vi "Main VI FTP FILE MANAGER.vi"() -> ()   [LabVIEW 2011]
doc: "FILE Archive & FTP is a software used to handle the file management of remote field sites using the HTI Data Logger or ATR series acoustic equipment that generates *.RAT and *.ATL files. The software monitors a specific folder on the local machine that the HTI equipment has been set up to move completed files of these types into. All other file types are ignored. The software continues to scan this file until a new file is added to the directory, on the addition of a file the NODE ARCHIVE & FTP software moves the file into an Archive directory (and if specified into a redundant Archive directory) then creates a *.ZIP version of the file and retains a copy of it in the Archive directory as well. All Zip files are then copied to a specified FTP host.\n\nNODE ARCHIVE & FTP will not try and move files for the last five minutes of an hour, or for the first five to ten minutes of the hour (based on CPU time). This is to allow the HTI hardware time to move all files at the top of the hour and avoid conflict. During the rest of the hour the software will continue to scan for new files. At any time a user can force a scan or FTP move by selecting the Manual Force FTP button or the Manual Archive Files button.\n\nNODE ARCHIVE & FTP creates an .INI file and a .CSV file in the programs application directory. The .INI file retains the last values of the file directory and FTP credentials used. The .CSV retains a history of *.ZIP files moved to the FTP and the status of their move, if there were errors or not. NODE ARCHIVE & FTP will continue to try and send the file to the FTP host until that file has completed the process with no errors. DO NOT remove or edit the .CSV file or the software will try and move all files up to the FTP again and will slow down the FTP Host."
uses:
  Controls/FTP Credintials.ctl
  Controls/File Management.ctl
  Controls/File Path directories.ctl
  Controls/Ping address and email notify.ctl
  Controls/PingElements.ctl
  SubVIs/Bini ArchiveAndFtpCluster.ctl
  <vilib>/Utility/sysdir.llb/System Directory Type.ctl
panel:
  in  "SaveConfig":bool
  in  "Settings":bool
  in  "Contacts":bool
  in  "Errors":bool
  in  "SetPingStats":bool
  in  "Addresses to Ping":T1
  in  "File type Cover":bool
  in  "Auto Archive":bool
  in  "Auto FTP":bool
  in  "update extentions":bool
  in  "ShutDown":bool
  in  "FTP Creds":T2={"Host"="", "UserName"="", "PassWord"="", "FTP File Path"="", "Timeout (S)"=0, "ActivePasive"=FALSE, "Binary Ascii"=FALSE, "Remote Port"=21} {"Timeout (S)" min=0 max=300 step=1}
  in  "SITE ID":string="Site Not Configured" caption="Site ID:"
  in  "File Management":T3
  in  "Manual FTP":bool
  out "Archive in progress":bool caption="Archive"
  out "Status FTP move":bool caption="FTP"
  in  "Manual Archive":bool
  in  "File output directories":T4={"Archive Location"=path "", "Archive Location 2"=path "<Not A Path>", "OutPut Path"=path "", "Directory(s) To Scan Files"=[]}
  in  "time date mod":bool
  out "Elapsed Time (H)":dbl caption="Time since Last File \nSize Check (H)" format="%#_3f"
  in  "recipients":string[](array[string])=["nmswyers@gmail.com"] caption="Errors & Warnings Email Recipients"
  out "hours":u8
  out "Email Notification Cluster":T5
  in  "shutting down closeout":bool
  in  "Time DaY":timestamp
  # "D\nI\nR\nE\nC\nT\nO\nR\nY\n\nS\nE\nT"
  # "FILE \n\nHANDLE\n\nMETHODS"
  # "FTP\n\nSETUP"
  # "Passive"
  # "Active"
  # "Binary"
  # "Ascii"
  # "File Handling Method"
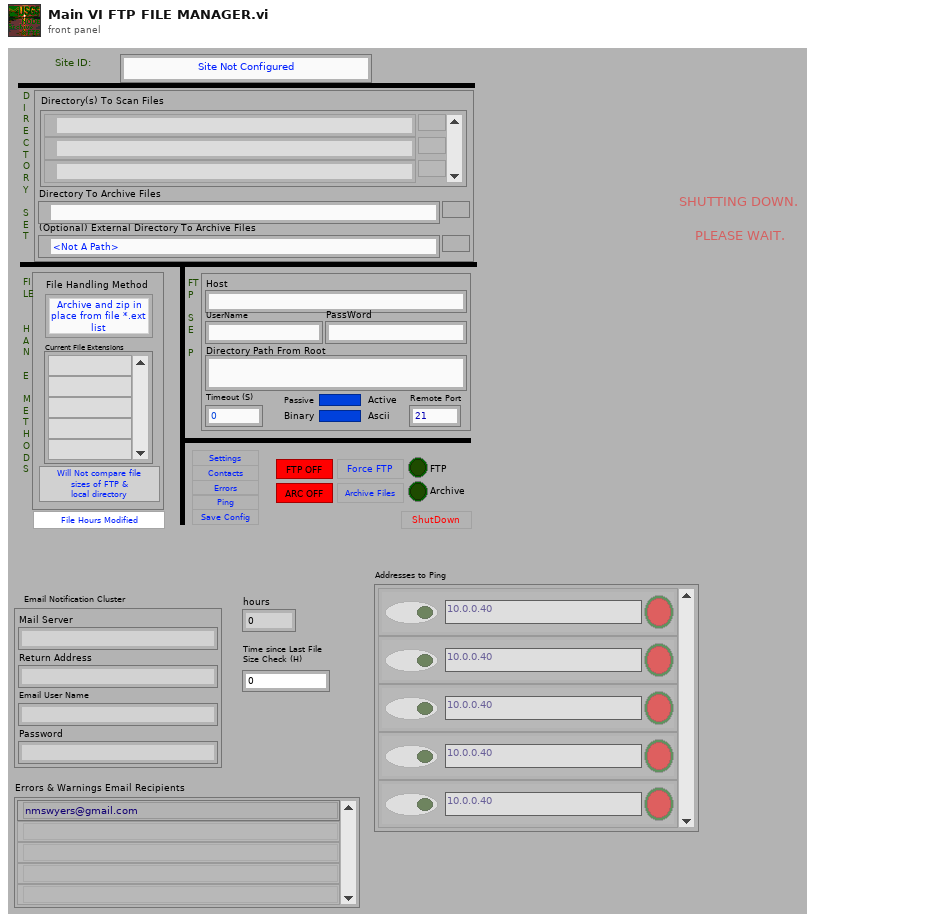
[diagram p1: front panel]
types:
  T1 = typedef "PingElements.ctl" = cluster{"AddressNode 1":string, "Response 1":bool, "Ping on Address 1":bool}[]
  T2 = typedef "FTP Credintials.ctl" = cluster{"Host":string, "UserName":string, "PassWord":string, "FTP File Path":string, "Timeout (S)":i32, "ActivePasive":bool, "Binary Ascii":bool, "Remote Port":u16}
  T3 = typedef "File Management.ctl" = cluster{"Comp File Size":bool, "File Handle Method":enum16{"Archive and zip in place from file *.ext list", "Archive and zip ALL file Types to archive directory", "Archive and zip to archive directory from file *.ext list", "Perform no file management"}, "file extention list":string[]}
  T4 = typedef "File Path directories.ctl" = cluster{"Archive Location":path, "Archive Location 2":path, "OutPut Path":path, "Directory(s) To Scan Files":path[]}
  T5 = typedef "Ping address and email notify.ctl" = cluster{"Mail Server":string, "Return Address":string, "Email User Name":string, "Password":string}
  T6 = enum16{"open", "replace", "create", "open or create", "replace or create", "replace or create with confirmation"}
  T7 = enum8{"Enabled", "Disabled", "Disabled and Grayed Out"}
  T8 = typedef "Bini ArchiveAndFtpCluster.ctl" = cluster{"Site ID":string, "File Management cluster":T3, "time stamp":timestamp, "File output directories":T4, "Auto FTP":bool, "Auto Archive":bool, "FTP CRED Cluster":T2, "hours old date mod(hours)":u8, "Email Notification Cluster":T5, "Email Recipiant List":string[], "Addresses to Ping":T1}
  T9 = enum16{"Archive and zip in place from file *.ext list", "Archive and zip ALL file Types to archive directory", "Archive and zip to archive directory from file *.ext list", "Perform no file management"}
  T10 = enum32{"Invalid", "Standard", "Closed", "Hidden", "Minimized", "Maximized"}
  T11 = cluster{"AddressNode 1":string, "Response 1":bool, "Ping on Address 1":bool}
  T12 = enum32{"invalid app kind", "Development System", "Run Time System", "Student Edition", "Embedded LabVIEW", "Evaluation", "Custom"}
  T13 = typedef "System Directory Type.ctl" = i32
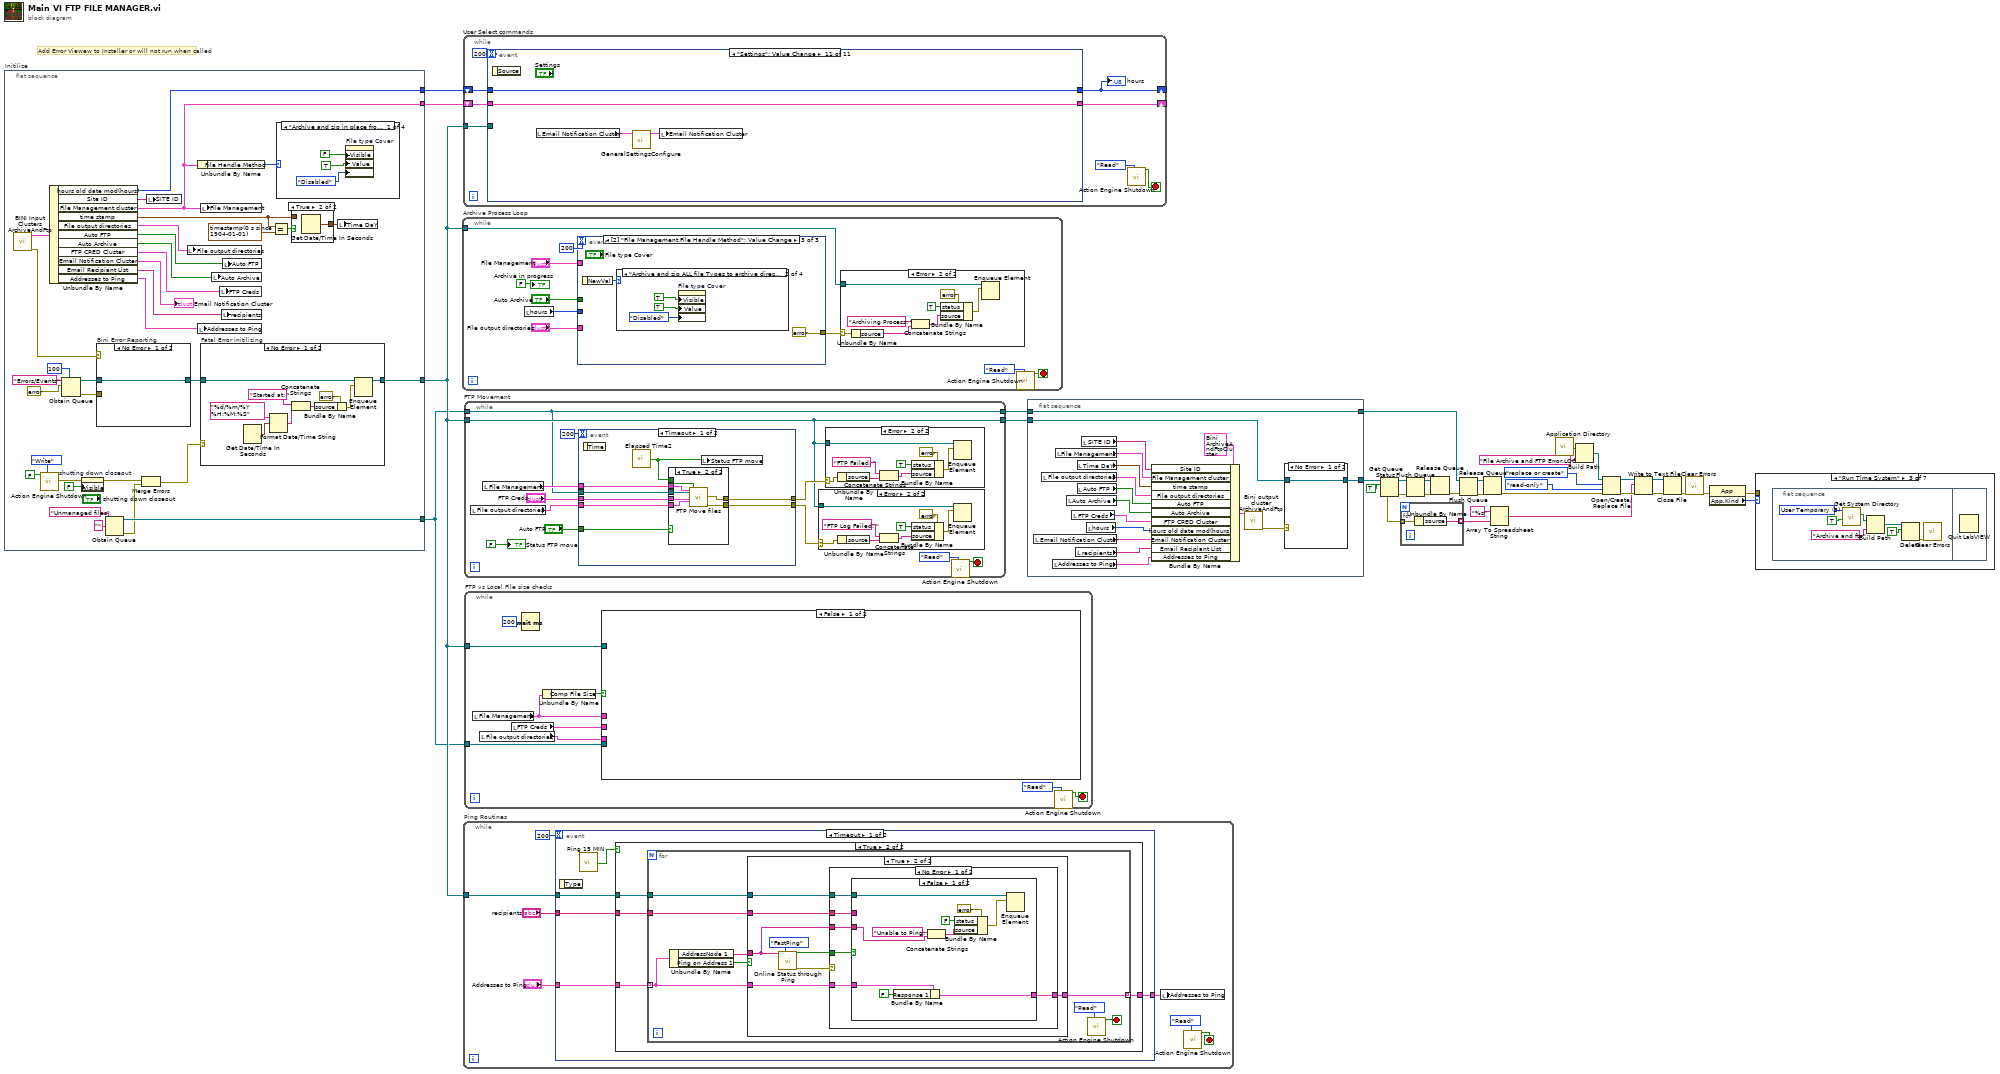
[diagram p0: block diagram]
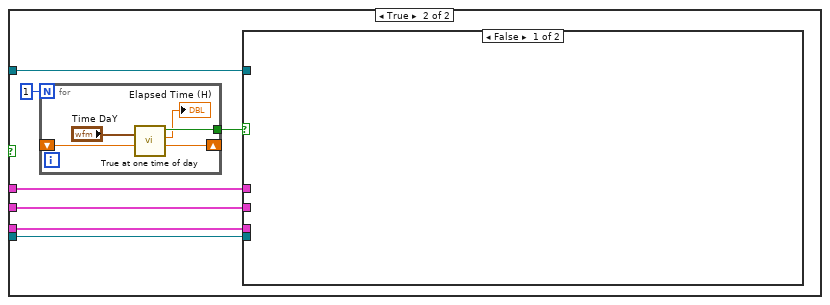
[diagram p2: hidden frame]
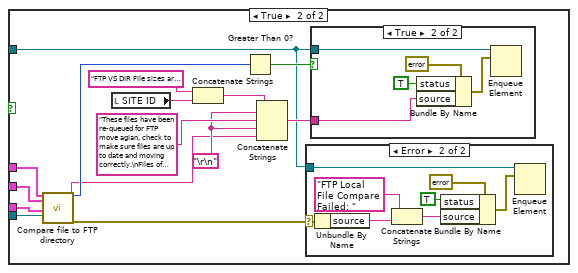
[diagram p3: hidden frame]
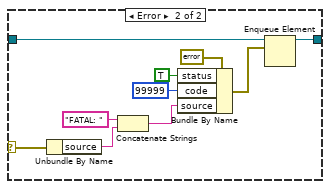
[diagram p7: hidden frame]
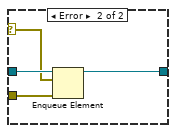
[diagram p8: hidden frame]
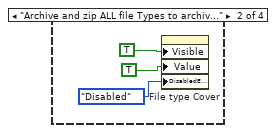
[diagram p9: hidden frame]
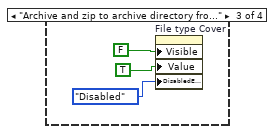
[diagram p10: hidden frame]
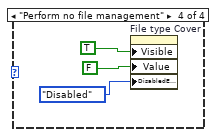
[diagram p11: hidden frame]
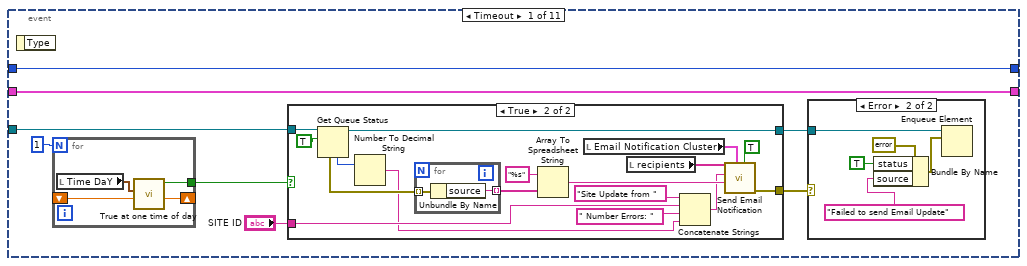
[diagram p12: hidden frame]
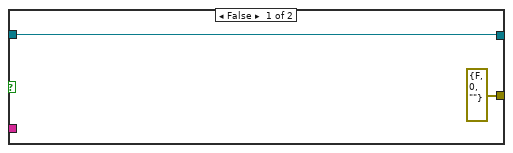
[diagram p14: hidden frame]
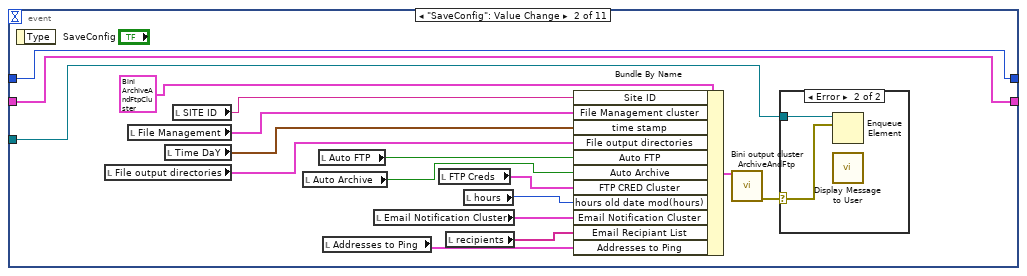
[diagram p15: hidden frame]
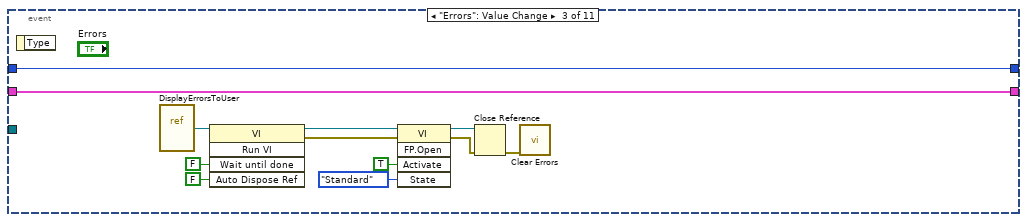
[diagram p17: hidden frame]
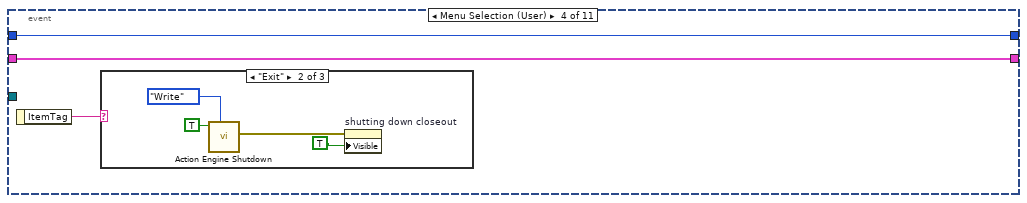
[diagram p18: hidden frame]
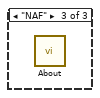
[diagram p20: hidden frame]
diagram:
  # "Add Error Viewew to Installer or will not run when called"
  n1 = flat-sequence "Initilize" {
    tunnel: [w66] -> w28
    tunnel: [w56] -> w31
    tunnel: [w51] -> w30
    tunnel: [w39] -> w29
    frame #0 {
      n2 = call "BINI Input Clusters ArchiveAndFtp.vi"() -> ("Bini Error out"=w46:errorcluster, "Bini Load"=w57:T8)  [unwired: 10 in]
      n3 = call "Action Engine Shutdown.vi"("Shutdown"=enum16{"Write", "Read"}."Write", "Shutdown (True to Shutdown)"=FALSE) -> ("error out"=w62:errorcluster)  [unwired: 8 in, 1 out]
      n4 = Unbundle By Name(w57) -> ("hours old date mod(hours)"=w51:u8, "Site ID"=w55:string, "File Management cluster"=w56:T3, "time stamp"=w35:timestamp, "File output directories"=w54:T4, "Auto FTP"=w53:bool, "Auto Archive"=w52:bool, "FTP CRED Cluster"=w50:T2, "Email Notification Cluster"=→"Email Notification Cluster":T5, "Email Recipiant List"=w48:string[], "Addresses to Ping"=w47:T1)
      n5 = Obtain Queue(max queue size (-1, unlimited)=100, name (unnamed)="Errors/Events", element data type=errorcluster {"status"=FALSE, "code"=0, "source"=""} ("error constant")) -> (queue out=w45:refnum<queue>, error out=w43:errorcluster)  [unwired: 2 in, 1 out]
      n6 = property on="shutting down closeout" class="Bool"(error in=w62, "Visible"=FALSE) -> (error out=w42:errorcluster)  [unwired: 1 in, 1 out]
      n7 = case "Bini Error Reporting" shown="No Error" w46 {
        selector: w46 -> [_ w92]
        tunnel: w45 -> [w90 w94]
        tunnel: [w90 w93] -> w40
        tunnel: w43 -> [_ w91]
        frame No Error {
        }
        frame Error {
          n8 = Enqueue Element(queue=w94, element=w92, error in (no error)=w91) -> (queue out=w93:refnum<queue>)  [unwired: 1 in, 2 out]
        }
      }
      n9 = Obtain Queue(name (unnamed)="Unmanaged files", element data type="" ("name (unnamed)")) -> (queue out=w66:refnum<queue>, error out=w60:errorcluster)  [unwired: 3 in, 1 out]
      n10 = Merge Errors(w42, w60) -> (w41:errorcluster)
      n11 = local write "SITE ID"(w55) -> ()
      n12 = local write "File output directories"(w54) -> ()
      n13 = Unbundle By Name(w56) -> ("File Handle Method"=w61:T9)
      n14 = local write "Addresses to Ping"(w47) -> ()
      n15 = local write "File Management"(w56) -> ()
      n16 = case "Fatal Error initilizing" shown="No Error" w41 {
        selector: w41 -> [_ w83]
        tunnel: w40 -> [w79 w89]
        tunnel: [w78 w88] -> w39
        frame No Error {
          n17 = Get Date/Time In Seconds() -> (seconds since 1Jan1904=w73:timestamp)
          n18 = Format Date/Time String(time format string (%c)="%d/%m/%Y %H:%M:%S", seconds (now)=w73) -> (date/time string=w72:string)  [unwired: 1 in]
          n19 = Concatenate Strings("Started at: " ("string"), w72) -> (w75:string)
          n20 = Bundle By Name(cluster=errorcluster {"status"=FALSE, "code"=0, "source"=""} ("element"), "source"=w75) -> (w76:errorcluster)
          n21 = Enqueue Element(queue=w79, element=w76) -> (queue out=w78:refnum<queue>)  [unwired: 2 in, 2 out]
        }
        frame Error {
          n22 = Unbundle By Name(w83) -> ("source"=w82:string)
          n23 = Concatenate Strings("FATAL: " ("string"), w82) -> (w85:string)
          n24 = Bundle By Name(cluster=errorcluster {"status"=FALSE, "code"=0, "source"=""} ("error constant"), "status"=TRUE, "code"=99999, "source"=w85) -> (w80:errorcluster)
          n25 = Enqueue Element(queue=w89, element=w80) -> (queue out=w88:refnum<queue>)  [unwired: 2 in, 2 out]
        }
      }
      n26 = local write "Auto Archive"(w52) -> ()
      n27 = local write "FTP Creds"(w50) -> ()
      n28 = local write "recipients"(w48) -> ()
      n29 = local write "Auto FTP"(w53) -> ()
      n30 = Equal?(x=w35, y=timestamp(0 s since 1904-01-01)) -> (x = y?=w38:bool)
      n31 = case shown="\"Archive and zip in place from file *.ext list\", Default" w61 {
        frame "Archive and zip in place from file *.ext list", Default {
          n32 = property on="File type Cover" class="Bool (strict)"("Visible"=FALSE, "Value"=TRUE ("File type Cover"), "DisabledEnum"=T7."Disabled" ("Disabled")) -> ()  [unwired: 2 in, 2 out]
        }
        frame "Archive and zip ALL file Types to archive directory" {
          n33 = property on="File type Cover" class="Bool (strict)"("Visible"=TRUE, "Value"=TRUE ("File type Cover"), "DisabledEnum"=T7."Disabled" ("Disabled")) -> ()  [unwired: 2 in, 2 out]
        }
        frame "Archive and zip to archive directory from file *.ext list" {
          n34 = property on="File type Cover" class="Bool (strict)"("Visible"=FALSE, "Value"=TRUE ("File type Cover"), "DisabledEnum"=T7."Disabled" ("Disabled")) -> ()  [unwired: 2 in, 2 out]
        }
        frame "Perform no file management" {
          n35 = property on="File type Cover" class="Bool (strict)"("Visible"=TRUE, "Value"=FALSE ("File type Cover"), "DisabledEnum"=T7."Disabled" ("Disabled")) -> ()  [unwired: 2 in, 2 out]
        }
      }
      n36 = case shown="True" w38 {
        tunnel: [w69 w70] -> w36
        tunnel: w35 -> [w69 _]
        frame False {
        }
        frame True {
          n37 = Get Date/Time In Seconds() -> (seconds since 1Jan1904=w70:timestamp)
        }
      }
      n38 = local write "Time DaY"(w36) -> ()
    }
  }
  n39 = while "Archive Process Loop" {
    tunnel: w29 -> [w107]
    stop <- w111 stop-if-true
    n40 = local read "hours"() -> (w108:u8)
    n41 = event shown="[2] \"File Management.File Handle Method\": Value Change" {
      selector: _ -> [_ _ _]
      dyn-events: _ -> [_ _ _]
      timeout: 200 -> [_ _ _]
      tunnel: [w130 w143 errorcluster {"status"=FALSE, "code"=0, "source"=""} ("error IO")] -> w110
      tunnel: "File output directories" -> [w125 w142 _]
      tunnel: "File Management" -> [w128 w140 _]
      tunnel: "Auto Archive" -> [w129 _ _]
      tunnel: w108 -> [w126 w139 _]
      event Timeout {
        n42 = event-data() -> ()  [unwired: 1 in, 1 out]
        n43 = call "Elapsed Time"() -> ("Time has Elapsed"=w127:bool)  [unwired: 12 in, 7 out]
        n44 = case shown="True" w129 {
          tunnel: w125 -> [w131 w138]
          tunnel: [errorcluster {"status"=FALSE, "code"=0, "source"=""} ("error IO") w137] -> w130
          tunnel: w128 -> [_ w136]
          tunnel: w127 -> [_ w135]
          tunnel: w126 -> [_ w134]
          tunnel: [w131 w133] -> _
          frame False {
          }
          frame True {
            n45 = call "Archive files move dir.vi"("hours old date mod(hours)"=w134, "File path input cluster"=w138, "File Management"=w136, "Timing True to archive"=w135) -> ("error IO"=w137:errorcluster, "File path input cluster (out)"=w133:T4)  [unwired: 4 in]
          }
        }
        n46 = local write "Archive in progress"(w127) -> ()
      }
      event "Manual Archive": Value Change {
        w141 = TRUE ("Status File move")
        n47 = event-data() -> ()  [unwired: 1 in, 1 out]
        n48 = local write "Archive in progress"(w141) -> ()
        n49 = call "Archive files move dir.vi"("hours old date mod(hours)"=w139, "File path input cluster"=w142, "File Management"=w140, "Timing True to archive"=w141) -> ("error IO"=w143:errorcluster)  [unwired: 4 in, 1 out]
      }
      event Value Change {
        n50 = event-data() -> ("NewVal"=w145:T9)  [unwired: 1 in]
        n51 = case shown="\"Archive and zip ALL file Types to archive directory\"" w145 {
          frame "Archive and zip in place from file *.ext list", Default {
            n52 = property on="File type Cover" class="Bool (strict)"("Visible"=FALSE, "Value"=TRUE ("File type Cover"), "DisabledEnum"=T7."Disabled" ("Disabled")) -> ()  [unwired: 2 in, 2 out]
          }
          frame "Archive and zip ALL file Types to archive directory" {
            n53 = property on="File type Cover" class="Bool (strict)"("Visible"=TRUE, "Value"=TRUE ("File type Cover"), "DisabledEnum"=T7."Disabled" ("Disabled")) -> ()  [unwired: 2 in, 2 out]
          }
          frame "Archive and zip to archive directory from file *.ext list" {
            n54 = property on="File type Cover" class="Bool (strict)"("Visible"=FALSE, "Value"=TRUE ("File type Cover"), "DisabledEnum"=T7."Disabled" ("Disabled")) -> ()  [unwired: 2 in, 2 out]
          }
          frame "Perform no file management" {
            n55 = property on="File type Cover" class="Bool (strict)"("Visible"=TRUE, "Value"=FALSE ("File type Cover"), "DisabledEnum"=T7."Disabled" ("Disabled")) -> ()  [unwired: 2 in, 2 out]
          }
        }
      }
    }
    n56 = case shown="Error" w110 {
      selector: w110 -> [_ w119]
      tunnel: w107 -> [_ w124]
      frame No Error {
      }
      frame Error {
        n57 = Unbundle By Name(w119) -> ("source"=w118:string)
        n58 = Concatenate Strings("Archiving Process: " ("string"), w118) -> (w117:string)
        n59 = Bundle By Name(cluster=errorcluster {"status"=FALSE, "code"=0, "source"=""} ("error constant"), "status"=TRUE, "source"=w117) -> (w122:errorcluster)
        n60 = Enqueue Element(queue=w124, element=w122) -> ()  [unwired: 2 in, 3 out]
      }
    }
    n61 = call "Action Engine Shutdown.vi"("Shutdown"=enum16{"Write", "Read"}."Read") -> ("Shutdown"=w111:bool)  [unwired: 9 in, 1 out]
    "Archive in progress" <- FALSE ("Archive in progress")
  }
  n62 = while "User Select commands" {
    shift-right: [w161] -> _
    shift-left: w30 -> [w162]
    shift-right: [w159] -> _
    shift-left: w31 -> [w160]
    tunnel: w29 -> [w158]
    stop <- w163 stop-if-true
    n63 = event shown="[10] \"Settings\": Value Change" {
      selector: _ -> [_ _ _ _ _ _ _ _ _ _ _]
      dyn-events: _ -> [_ _ _ _ _ _ _ _ _ _ _]
      timeout: 200 -> [_ _ _ _ _ _ _ _ _ _ _]
      tunnel: w162 -> [w173 w207 w234 w236 w243 w251 w257 w264 w282 w290 w294]
      tunnel: [w173 w207 w234 w236 w243 w251 w257 w263 w282 w290 w294] -> w161
      tunnel: w160 -> [w172 w206 w233 w235 w242 w250 w256 w262 w285 w289 w293]
      tunnel: [w172 w206 w233 w235 w242 w250 w256 w262 w283 w289 w293] -> w159
      tunnel: w158 -> [w168 w204 _ _ _ _ _ _ _ _ _]
      event Timeout {
        n64 = event-data() -> ()  [unwired: 1 in, 1 out]
        n65 = for {
          N: 1 -> [_]
          tunnel: [w203] -> w171
          shift-right: [w202] -> _
          shift-left: _ -> [w201]
          n66 = local read "Time DaY"() -> (w200:timestamp)
          n67 = call "True at one time of day.vi"("Next start time in"=w201, "Time stamp from INI (only will use time Not date)"=w200) -> ("next start time out"=w202:dbl, "Time has Elapsed"=w203:bool)  [unwired: 6 in, 2 out]
        }
        n68 = case shown="True" w171 {
          tunnel: "SITE ID" -> [_ w185]
          tunnel: w168 -> [w179 w193]
          tunnel: [errorcluster {"status"=FALSE, "code"=0, "source"=""} ("error out") w194] -> w167
          tunnel: [w179 w181] -> w166
          frame False {
          }
          frame True {
            n69 = Get Queue Status(queue=w193, return elements? (F)=TRUE) -> (queue out=w181:refnum<queue>, # elements in queue=w184:i32, elements=w191:errorcluster[])  [unwired: 1 in, 5 out]
            n70 = Number To Decimal String(number=w184) -> (decimal integer string=w182:string)  [unwired: 1 in]
            n71 = for {
              tunnel: w191 -> [w199] mode=indexing
              tunnel: [w198] -> w190 mode=indexing
              n72 = Unbundle By Name(w199) -> ("source"=w198:string)
            }
            n73 = Array To Spreadsheet String(array=w190, 3:"%s" ("format string")) -> (spreadsheet string=w188:string)  [unwired: 1 in]
            n74 = local read "Email Notification Cluster"() -> (w195:T5)
            n75 = local read "recipients"() -> (w197:string[])
            n76 = Concatenate Strings("Site Update from " ("string"), w185, " Number Errors: " ("string"), w182) -> (w187:string)
            n77 = call "Send Email Notification.vi"("Send Email Notification"=TRUE, "Email Notification Cluster (in)"=w195, "message"=w188, "Email Subject"=w187, "recipients"=w197) -> ("error out"=w194:errorcluster)  [unwired: 6 in]
          }
        }
        n78 = case shown="Error" w167 {
          tunnel: w166 -> [_ w178]
          frame No Error {
          }
          frame Error {
            n79 = Bundle By Name(cluster=errorcluster {"status"=FALSE, "code"=0, "source"=""} ("error constant"), "status"=TRUE, "source"="Failed to send Email Update") -> (w176:errorcluster)
            n80 = Enqueue Element(queue=w178, element=w176) -> ()  [unwired: 2 in, 3 out]
          }
        }
      }
      event "SaveConfig": Value Change {
        n81 = event-data() -> ()  [unwired: 1 in, 1 out]
        n82 = local read "File output directories"() -> (w213:T4)
        n83 = local read "File Management"() -> (w211:T3)
        n84 = local read "Time DaY"() -> (w212:timestamp)
        n85 = local read "SITE ID"() -> (w210:string)
        n86 = local read "Auto Archive"() -> (w215:bool)
        n87 = local read "Auto FTP"() -> (w214:bool)
        n88 = local read "Addresses to Ping"() -> (w220:T1)
        n89 = local read "Email Notification Cluster"() -> (w218:T5)
        n90 = local read "FTP Creds"() -> (w216:T2)
        n91 = local read "recipients"() -> (w219:string[])
        n92 = local read "hours"() -> (w217:u8)
        n93 = Bundle By Name(cluster=T8 {"Site ID"="", "File Management cluster"={"Comp File Size"=FALSE, "File Handle Method"=enum."Archive and zip in place from file *.ext list", "file extention list"=[]}, "time stamp"=timestamp(0 s since 1904-01-01), "File output directories"={"Archive Location"=path "", "Archive Location 2"=path "<Not A Path>", "OutPut Path"=path "", "Directory(s) To Scan Files"=[]}, "Auto FTP"=FALSE, "Auto Archive"=FALSE, "FTP CRED Cluster"={"Host"="", "UserName"="", "PassWord"="", "FTP File Path"="", "Timeout (S)"=60, "ActivePasive"=FALSE, "Binary Ascii"=FALSE, "Remote Port"=0}, "hours old date mod(hours)"=2, "Email Notification Cluster"={"Mail Server"="", "Return Address"="", "Email User Name"="", "Password"=""}, "Email Recipiant List"=[], "Addresses to Ping"=[]} ("Settings To Bini"), "Site ID"=w210, "File Management cluster"=w211, "time stamp"=w212, "File output directories"=w213, "Auto FTP"=w214, "Auto Archive"=w215, "FTP CRED Cluster"=w216, "hours old date mod(hours)"=w217, "Email Notification Cluster"=w218, "Email Recipiant List"=w219, "Addresses to Ping"=w220) -> (w209:T8)
        n94 = call "Bini output cluster ArchiveAndFtp.vi"("Settings To Bini"=w209) -> ("Bini Error out"=w205:errorcluster)  [unwired: 14 in]
        n95 = case shown="Error" w205 {
          selector: w205 -> [_ w221]
          tunnel: w204 -> [_ w222]
          frame No Error {
          }
          frame Error {
            n96 = Enqueue Element(queue=w222, element=w221) -> ()  [unwired: 2 in, 3 out]
            n97 = call "Display Message to User"() -> ()  [unwired: 10 in, 2 out]
          }
        }
      }
      event "Errors": Value Change {
        n98 = event-data() -> ()  [unwired: 1 in, 1 out]
        n99 = vi-ref "DisplayErrorsToUser.vi"() -> (w223:refnum<vi>)
        n100 = invoke class="VI" method="Run VI"(reference=w223, "Wait until done"=FALSE ("Wait Until Done"), "Auto Dispose Ref"=FALSE ("Auto Dispose Reference")) -> (reference out=w230:refnum<vi>, error out=w229:errorcluster)  [unwired: 2 in, 3 out]
        n101 = invoke class="VI" method="FP.Open"(reference=w230, error in=w229, "Activate"=TRUE ("Activate?"), "State"=T10."Standard") -> (reference out=w226:refnum<vi>, error out=w225:errorcluster)  [unwired: 1 in, 3 out]
        n102 = Close Reference(reference=w226, error in (no error)=w225) -> (error out=w224:errorcluster)
        n103 = call <vilib>:"Clear Errors.vi"("error in (no error)"=w224) -> ()  [unwired: 6 in, 1 out]
      }
      event Menu Selection (User) {
        n104 = event-data() -> ("ItemTag"=w237:string)  [unwired: 1 in]
        n105 = case shown="\"Exit\"" w237 {
          frame "Null", Default {
          }
          frame "Exit" {
            n106 = call "Action Engine Shutdown.vi"("Shutdown"=enum16{"Write", "Read"}."Write", "Shutdown (True to Shutdown)"=TRUE ("Stop Button")) -> ("error out"=w238:errorcluster)  [unwired: 8 in, 1 out]
            n107 = property on="shutting down closeout" class="Bool"(error in=w238, "Visible"=TRUE) -> ()  [unwired: 1 in, 2 out]
          }
          frame "NAF" {
            n108 = call "About.vi"() -> ()  [unwired: 12 in]
          }
        }
      }
      event "ShutDown": Value Change {
        n109 = event-data() -> ()  [unwired: 1 in, 1 out]
        n110 = Two Button Dialog(message="Are you sure you want to shut down the software? This will end all file management of the Archive directories and FTP file movement until the software is restarted.\nIf the Archiving In Progress, or the FTP In Progress is lit the software will shut down as soon as the process is done.", 2:"Shutdown" ("T button name (\"OK\")")) -> (T button?=w246:bool)  [unwired: 1 in]
        n111 = case shown="True" w246 {
          frame False {
          }
          frame True {
            n112 = property on="shutting down closeout" class="Bool"("Visible"=TRUE) -> ()  [unwired: 2 in, 2 out]
            n113 = call "Action Engine Shutdown.vi"("Shutdown"=enum16{"Write", "Read"}."Write", "Shutdown (True to Shutdown)"=TRUE) -> ()  [unwired: 8 in, 2 out]
          }
        }
      }
      event Application Instance Close? {
        w255 = TRUE ("SilentShutdown")
        n114 = event-data() -> ()  [unwired: 1 in, 1 out]
        n115 = call "Action Engine Shutdown.vi"("Shutdown"=enum16{"Write", "Read"}."Write", "Shutdown (True to Shutdown)"=TRUE) -> ()  [unwired: 8 in, 2 out]
        n116 = property on="shutting down closeout" class="Bool"("Visible"=TRUE) -> ()  [unwired: 2 in, 2 out]
        n117 = event-data("SilentShutdown"=w255, "Discard?"=w255) -> ()  [unwired: 1 in, 1 out]
      }
      event Panel Close? {
        n118 = event-data() -> ()  [unwired: 1 in, 1 out]
        n119 = call "Action Engine Shutdown.vi"("Shutdown"=enum16{"Write", "Read"}."Write", "Shutdown (True to Shutdown)"=TRUE) -> ()  [unwired: 8 in, 2 out]
        n120 = property on="shutting down closeout" class="Bool"("Visible"=TRUE) -> ()  [unwired: 2 in, 2 out]
        n121 = event-data("Discard?"=TRUE) -> ()  [unwired: 1 in, 1 out]
      }
      event "time date mod": Value Change {
        n122 = event-data() -> ()  [unwired: 1 in, 1 out]
        n123 = Number To Decimal String(number=w264) -> (decimal integer string=w272:string)  [unwired: 1 in]
        n124 = Concatenate Strings("The Current number of hours that need to passed on a files last modified date before the file will be archived and moved to the ftp server." ("Message"), "\r\n", w272) -> (w270:string)
        n125 = call "Display Message to User2"("Message"=w270) -> ("error out"=w267:errorcluster, "Change Value"=w268:bool)  [unwired: 9 in]
        n126 = call "Prompt User for Input2"("Enable"=w268, "error in (no error)"=w267) -> ("(Hours)"=w266:dbl, "OK"=w265:bool, "error out"=w273:errorcluster)  [unwired: 15 in]
        n127 = case shown="No Error" w273 {
          tunnel: w265 -> [w277 _]
          tunnel: w266 -> [w276 _]
          tunnel: [w275 w281] -> w263
          tunnel: w264 -> [w274 w281]
          frame No Error {
            n128 = case shown="True" w277 {
              tunnel: w276 -> [_ w280]
              tunnel: w274 -> [w278 _]
              tunnel: [w278 w279] -> w275
              frame False {
              }
              frame True {
                n129 = To Unsigned Byte Integer(number=w280) -> (unsigned 8bit integer=w279:u8)
              }
            }
          }
          frame Error {
          }
        }
      }
      event "update extentions": Value Change {
        n130 = event-data() -> ()  [unwired: 1 in, 1 out]
        n131 = Unbundle By Name(w285) -> ("file extention list"=w284:string[])
        n132 = call "Flie Extention list.vi"("file extention list IN"=w284) -> ("File extention list (out)"=w286:string[])  [unwired: 10 in]
        n133 = Bundle By Name(cluster=w285, "file extention list"=w286) -> (w283:T3)
        n134 = local write "File Management"(w283) -> ()
      }
      event "Contacts": Value Change {
        n135 = event-data() -> ()  [unwired: 1 in, 1 out]
        n136 = local read "recipients"() -> (w288:string[])
        n137 = call "SetContactList.vi"("recipients IN"=w288) -> ("recipients OUT"=w287:string[])  [unwired: 10 in]
        n138 = local write "recipients"(w287) -> ()
      }
      event "Settings": Value Change {
        n139 = event-data() -> ()  [unwired: 1 in, 1 out]
        n140 = local read "Email Notification Cluster"() -> (w292:T5)
        n141 = call "GeneralSettingsConfigure.vi"("Email Notification Cluster in"=w292) -> ("Email Notification Cluster out"=w291:T5)  [unwired: 10 in]
        n142 = local write "Email Notification Cluster"(w291) -> ()
      }
    }
    "hours" <- w161
    n143 = call "Action Engine Shutdown.vi"("Shutdown"=enum16{"Write", "Read"}."Read") -> ("Shutdown"=w163:bool)  [unwired: 9 in, 1 out]
  }
  n144 = while "Ping Routines" {
    tunnel: w29 -> [w297]
    stop <- w298 stop-if-true
    n145 = event shown="[0] Timeout" {
      selector: _ -> [_ _]
      dyn-events: _ -> [_ _]
      timeout: 200 -> [_ _]
      tunnel: "recipients" -> [w305 _]
      tunnel: "Addresses to Ping" -> [w304 w364]
      tunnel: w297 -> [w303 _]
      tunnel: [w302 w363] -> w296
      event Timeout {
        n146 = event-data() -> ()  [unwired: 1 in, 1 out]
        n147 = call "Ping 15 MIN"() -> ("Time has Elapsed"=w306:bool)  [unwired: 12 in, 7 out]
        n148 = case shown="True" w306 {
          tunnel: w305 -> [_ w311]
          tunnel: w304 -> [w307 w310]
          tunnel: w303 -> [_ w309]
          tunnel: [w307 w308] -> w302
          frame False {
          }
          frame True {
            n149 = for {
              tunnel: w311 -> [w319]
              tunnel: w310 -> [w314] mode=indexing
              tunnel: w309 -> [w313]
              tunnel: [w312] -> w308 mode=indexing
              stop <- w316 stop-if-true
              n150 = Unbundle By Name(w314) -> ("AddressNode 1"=w315:string, "Ping on Address 1"=w318:bool)
              n151 = case shown="True" w318 {
                tunnel: w315 -> [_ w327]
                tunnel: w319 -> [_ w330]
                tunnel: w314 -> [w322 w328]
                tunnel: w313 -> [_ w324]
                tunnel: [w320 w323] -> w312
                frame False {
                  n152 = Bundle By Name(cluster=w322, "Response 1"=FALSE) -> (w320:T11)
                }
                frame True {
                  n153 = call "Online Status through Ping.vi"("AddressToPing"=w327, "Ping Method"=enum16{"LongPing", "NormalPing", "FastPing"}."FastPing") -> ("Connection?"=w329:bool, "error out"=w325:errorcluster)  [unwired: 9 in, 3 out]
                  n154 = case shown="No Error" w325 {
                    selector: w325 -> [_ w355]
                    tunnel: w330 -> [w336 _]
                    tunnel: w329 -> [w335 _]
                    tunnel: w328 -> [w334 w358]
                    tunnel: w327 -> [w333 w352]
                    tunnel: w324 -> [w332 w362]
                    tunnel: [w331 w356] -> w323
                    frame No Error {
                      n155 = case shown="False" w335 {
                        tunnel: w336 -> [_ _]
                        tunnel: w333 -> [w337 _]
                        tunnel: w334 -> [w346 w349]
                        tunnel: w332 -> [w343 _]
                        tunnel: [w345 w347] -> w331
                        frame False {
                          n156 = Bundle By Name(cluster=w346, "Response 1"=FALSE) -> (w345:T11)
                          n157 = Concatenate Strings("Unable to Ping: " ("string"), w337) -> (w339:string)
                          n158 = Bundle By Name(cluster=errorcluster {"status"=FALSE, "code"=0, "source"=""} ("error constant"), "status"=FALSE, "source"=w339) -> (w341:errorcluster)
                          n159 = Enqueue Element(queue=w343, element=w341) -> ()  [unwired: 2 in, 3 out]
                        }
                        frame True {
                          n160 = Bundle By Name(cluster=w349, "Response 1"=TRUE) -> (w347:T11)
                        }
                      }
                    }
                    frame Error {
                      n161 = Unbundle By Name(w355) -> ("source"=w350:string)
                      n162 = Bundle By Name(cluster=w358, "Response 1"=FALSE) -> (w356:T11)
                      n163 = Concatenate Strings("Ping Request Failed on IP: " ("string"), w352, " : " ("string"), w350) -> (w354:string)
                      n164 = Bundle By Name(cluster=errorcluster {"status"=FALSE, "code"=0, "source"=""} ("error constant"), "status"=TRUE, "source"=w354) -> (w360:errorcluster)
                      n165 = Enqueue Element(queue=w362, element=w360) -> ()  [unwired: 2 in, 3 out]
                    }
                  }
                }
              }
              n166 = call "Action Engine Shutdown.vi"("Shutdown"=enum16{"Write", "Read"}."Read") -> ("Shutdown"=w316:bool)  [unwired: 9 in, 1 out]
            }
          }
        }
      }
      event "SetPingStats": Value Change {
        n167 = event-data() -> ()  [unwired: 1 in, 1 out]
        n168 = call "SetPingAddresses.vi"("Addresses to Ping(in)"=w364) -> ("Addresses to Ping(out)"=w363:T1)  [unwired: 10 in]
      }
    }
    n169 = local write "Addresses to Ping"(w296) -> ()
    n170 = call "Action Engine Shutdown.vi"("Shutdown"=enum16{"Write", "Read"}."Read") -> ("Shutdown"=w298:bool)  [unwired: 9 in, 1 out]
  }
  n171 = while "FTP Movement" {
    tunnel: w28 -> [w365]
    tunnel: w29 -> [w366]
    tunnel: [w366] -> w27
    tunnel: [w365] -> w6
    stop <- w370 stop-if-true
    n172 = local read "File output directories"() -> (w374:T4)
    n173 = local read "File Management"() -> (w372:T3)
    n174 = event shown="[0] Timeout" {
      selector: _ -> [_ _]
      dyn-events: _ -> [_ _]
      timeout: 200 -> [_ _]
      tunnel: w365 -> [w400 w412]
      tunnel: [w399 w413] -> w368
      tunnel: [w398 w414] -> w367
      tunnel: "FTP Creds" -> [w397 w411]
      tunnel: w374 -> [w395 w409]
      tunnel: w372 -> [w396 w410]
      tunnel: "Auto FTP" -> [w394 _]
      event Timeout {
        n175 = event-data() -> ()  [unwired: 1 in, 1 out]
        n176 = call "Elapsed Time2"() -> ("Time has Elapsed"=w393:bool)  [unwired: 12 in, 7 out]
        n177 = case shown="True" w394 {
          tunnel: w393 -> [_ w408]
          tunnel: [w401 w407] -> w398
          tunnel: [w401 w406] -> w399
          tunnel: w400 -> [_ w405]
          tunnel: w396 -> [_ w404]
          tunnel: w397 -> [_ w403]
          tunnel: w395 -> [_ w402]
          frame False {
            w401 = errorcluster {"status"=FALSE, "code"=0, "source"=""} ("Log file write error condition")
          }
          frame True {
            n178 = call "FTP Move files.vi"("File Management"=w404, "Unmanaged Files Queue"=w405, "FTP Creds"=w403, "File output directories"=w402, "Timing true or false to zip files"=w408) -> ("Unmanaged files queue error out"=w406:errorcluster, "Log file write error condition"=w407:errorcluster)  [unwired: 12 in, 1 out]
          }
        }
        n179 = local write "Status FTP move"(w393) -> ()
      }
      event "Manual FTP": Value Change {
        n180 = event-data() -> ()  [unwired: 1 in, 1 out]
        n181 = local write "Status FTP move"(TRUE ("Status FTP move")) -> ()
        n182 = call "FTP Move files.vi"("File Management"=w410, "Unmanaged Files Queue"=w412, "FTP Creds"=w411, "File output directories"=w409, "Timing true or false to zip files"=TRUE) -> ("Unmanaged files queue error out"=w413:errorcluster, "Log file write error condition"=w414:errorcluster)  [unwired: 12 in, 1 out]
      }
    }
    n183 = case shown="Error" w367 {
      selector: w367 -> [_ w380]
      tunnel: w366 -> [_ w384]
      frame No Error {
      }
      frame Error {
        n184 = Unbundle By Name(w380) -> ("source"=w379:string)
        n185 = Concatenate Strings("FTP Log Failed: " ("string"), w379) -> (w378:string)
        n186 = Bundle By Name(cluster=errorcluster {"status"=FALSE, "code"=0, "source"=""} ("error constant"), "status"=TRUE, "source"=w378) -> (w382:errorcluster)
        n187 = Enqueue Element(queue=w384, element=w382) -> ()  [unwired: 2 in, 3 out]
      }
    }
    n188 = case shown="Error" w368 {
      selector: w368 -> [_ w388]
      tunnel: w366 -> [_ w392]
      frame No Error {
      }
      frame Error {
        n189 = Unbundle By Name(w388) -> ("source"=w387:string)
        n190 = Concatenate Strings("FTP Failed: " ("string"), w387) -> (w386:string)
        n191 = Bundle By Name(cluster=errorcluster {"status"=FALSE, "code"=0, "source"=""} ("error constant"), "status"=TRUE, "source"=w386) -> (w390:errorcluster)
        n192 = Enqueue Element(queue=w392, element=w390) -> ()  [unwired: 2 in, 3 out]
      }
    }
    n193 = call "Action Engine Shutdown.vi"("Shutdown"=enum16{"Write", "Read"}."Read") -> ("Shutdown"=w370:bool)  [unwired: 9 in, 1 out]
    "Status FTP move" <- FALSE ("Status FTP move")
  }
  n194 = while "FTP vs Local File size checks" {
    tunnel: w29 -> [w420]
    tunnel: w28 -> [w423]
    stop <- w418 stop-if-true
    n195 = local read "File Management"() -> (w425:T3)
    n196 = local read "File output directories"() -> (w422:T4)
    n197 = local read "FTP Creds"() -> (w421:T2)
    n198 = Wait (ms)(milliseconds to wait=u32 200) -> ()  [unwired: 1 out]
    n199 = Unbundle By Name(w425) -> ("Comp File Size"=w424:bool)
    n200 = case shown="False" w424 {
      tunnel: w425 -> [_ w430]
      tunnel: w423 -> [_ w429]
      tunnel: w422 -> [_ w428]
      tunnel: w421 -> [_ w427]
      tunnel: w420 -> [_ w426]
      frame False {
      }
      frame True {
        n201 = for {
          N: 1 -> [_]
          tunnel: [w436] -> w432
          shift-right: [w434] -> _
          shift-left: _ -> [w433]
          n202 = call "True at one time of day.vi"("Next start time in"=w433, "Time stamp from INI (only will use time Not date)"="Time DaY") -> ("next start time out"=w434:dbl, "Time Until Next Scan (H)"=→"Elapsed Time (H)":dbl, "Time has Elapsed"=w436:bool)  [unwired: 6 in, 1 out]
        }
        n203 = case shown="False" w432 {
          tunnel: w430 -> [_ w445]
          tunnel: w429 -> [_ w444]
          tunnel: w428 -> [_ w443]
          tunnel: w427 -> [_ w442]
          tunnel: w426 -> [_ w439]
          frame False {
          }
          frame True {
            w450 = "\r\n"
            n204 = call "Compare file to FTP directory.vi"("File Management"=w445, "FTP Creds"=w442, "File output directories"=w443, "Unmanaged Files Queue"=w444) -> ("number of unmached files"=w447:i32, "unmatched file names"=w446:string, "Unmanaged files queue error out"=w438:errorcluster)  [unwired: 12 in, 1 out]
            n205 = local read "SITE ID"() -> (w448:string)
            n206 = Concatenate Strings("FTP VS DIR File sizes are different: " ("string"), w448) -> (w449:string)
            n207 = Greater Than 0?(x=w447) -> (x > 0?=w441:bool)
            n208 = Concatenate Strings(w449, w450, "These files have been re-queued for FTP move agian, check to make sure files are up to date and moving correctly.\nFiles of issue are listed below.\n\nLIST:" ("string"), w450, w446) -> (w440:string)
            n209 = case shown="Error" w438 {
              selector: w438 -> [_ w455]
              tunnel: w439 -> [_ w460]
              frame No Error {
              }
              frame Error {
                n210 = Unbundle By Name(w455) -> ("source"=w454:string)
                n211 = Concatenate Strings("FTP Local File Compare Failed: " ("string"), w454) -> (w456:string)
                n212 = Bundle By Name(cluster=errorcluster {"status"=FALSE, "code"=0, "source"=""} ("error constant"), "status"=TRUE, "source"=w456) -> (w458:errorcluster)
                n213 = Enqueue Element(queue=w460, element=w458) -> ()  [unwired: 2 in, 3 out]
              }
            }
            n214 = case shown="True" w441 {
              tunnel: w439 -> [_ w465]
              tunnel: w440 -> [_ w461]
              frame False {
              }
              frame True {
                n215 = Bundle By Name(cluster=errorcluster {"status"=FALSE, "code"=0, "source"=""} ("error constant"), "status"=TRUE, "source"=w461) -> (w463:errorcluster)
                n216 = Enqueue Element(queue=w465, element=w463) -> ()  [unwired: 2 in, 3 out]
              }
            }
          }
        }
      }
    }
    n217 = call "Action Engine Shutdown.vi"("Shutdown"=enum16{"Write", "Read"}."Read") -> ("Shutdown"=w418:bool)  [unwired: 9 in, 1 out]
  }
  n218 = flat-sequence {
    tunnel: w27 -> [w468]
    tunnel: [w467] -> w26
    tunnel: w6 -> [w466]
    tunnel: [w466] -> w3
    frame #0 {
      n219 = local read "Email Notification Cluster"() -> (w472:T5)
      n220 = local read "File output directories"() -> (w477:T4)
      n221 = local read "Addresses to Ping"() -> (w470:T1)
      n222 = local read "File Management"() -> (w479:T3)
      n223 = local read "Auto Archive"() -> (w475:bool)
      n224 = local read "FTP Creds"() -> (w474:T2)
      n225 = local read "recipients"() -> (w471:string[])
      n226 = local read "Time DaY"() -> (w478:timestamp)
      n227 = local read "Auto FTP"() -> (w476:bool)
      n228 = local read "SITE ID"() -> (w480:string)
      n229 = local read "hours"() -> (w473:u8)
      n230 = Bundle By Name(cluster=T8 {"Site ID"="", "File Management cluster"={"Comp File Size"=FALSE, "File Handle Method"=enum."Archive and zip in place from file *.ext list", "file extention list"=[]}, "time stamp"=timestamp(0 s since 1904-01-01), "File output directories"={"Archive Location"=path "", "Archive Location 2"=path "<Not A Path>", "OutPut Path"=path "", "Directory(s) To Scan Files"=[]}, "Auto FTP"=FALSE, "Auto Archive"=FALSE, "FTP CRED Cluster"={"Host"="", "UserName"="", "PassWord"="", "FTP File Path"="", "Timeout (S)"=60, "ActivePasive"=FALSE, "Binary Ascii"=FALSE, "Remote Port"=0}, "hours old date mod(hours)"=2, "Email Notification Cluster"={"Mail Server"="", "Return Address"="", "Email User Name"="", "Password"=""}, "Email Recipiant List"=[], "Addresses to Ping"=[]} ("Settings To Bini"), "Site ID"=w480, "File Management cluster"=w479, "time stamp"=w478, "File output directories"=w477, "Auto FTP"=w476, "Auto Archive"=w475, "FTP CRED Cluster"=w474, "hours old date mod(hours)"=w473, "Email Notification Cluster"=w472, "Email Recipiant List"=w471, "Addresses to Ping"=w470) -> (w481:T8)
      n231 = call "Bini output cluster ArchiveAndFtp.vi"("Settings To Bini"=w481) -> ("Bini Error out"=w469:errorcluster)  [unwired: 14 in]
      n232 = case shown="No Error" w469 {
        selector: w469 -> [_ w485]
        tunnel: w468 -> [w483 w486]
        tunnel: [w483 w484] -> w467
        frame No Error {
        }
        frame Error {
          n233 = Enqueue Element(queue=w486, element=w485) -> (queue out=w484:refnum<queue>)  [unwired: 2 in, 2 out]
        }
      }
    }
  }
  n234 = Get Queue Status(queue=w26, return elements? (F)=TRUE) -> (queue out=w19:refnum<queue>, error out=w18:errorcluster, elements=w24:errorcluster[])  [unwired: 1 in, 5 out]
  n235 = for {
    tunnel: w24 -> [w488] mode=indexing
    tunnel: [w487] -> w23 mode=indexing
    n236 = Unbundle By Name(w488) -> ("source"=w487:string)
  }
  n237 = Flush Queue(queue=w19, error in (no error)=w18) -> (queue out=w21:refnum<queue>, error out=w20:errorcluster)  [unwired: 1 out]
  n238 = Release Queue(queue=w21, error in (no error)=w20) -> (error out=w4:errorcluster)  [unwired: 1 in, 2 out]
  n239 = Flush Queue(queue=w3, error in (no error)=w4) -> (queue out=w5:refnum<queue>, error out=w2:errorcluster)  [unwired: 1 out]
  n240 = Release Queue(queue=w5, error in (no error)=w2) -> (error out=w1:errorcluster)  [unwired: 1 in, 2 out]
  n241 = Array To Spreadsheet String(array=w23, 3:"%s" ("format string")) -> (spreadsheet string=w7:string)  [unwired: 1 in]
  n242 = call <vilib>:"Application Directory.vi"() -> ("Application Directory"=w16:path)
  n243 = Build Path(base path=w16, name or relative path="File Archive and FTP Error.LOG") -> (appended path=w13:path)
  n244 = Open/Create/Replace File(file path (use dialog)=w13, error in=w1, operation (0:open)=T6."replace or create", access (0:read/write)=enum16{"read/write", "read-only", "write-only"}."read-only") -> (refnum out=w14:refnum<file>, error out=w15:errorcluster)  [unwired: 2 in, 1 out]
  n245 = Write to Text File(file (use dialog)=w14, text=w7, error in=w15) -> (refnum out=w10:refnum<file>, error out=w9:errorcluster)  [unwired: 1 in, 1 out]
  n246 = Close File(refnum=w10, error in=w9) -> (error out=w8:errorcluster)  [unwired: 1 out]
  n247 = call <vilib>:"Clear Errors.vi"("error in (no error)"=w8) -> ("error out"=w32:errorcluster)  [unwired: 6 in]
  n248 = property class="App"(error in=w32) -> (error out=w33:errorcluster, "App.Kind"=w34:T12)  [unwired: 1 in, 1 out]
  n249 = case shown="\"Run Time System\"" w34 {
    tunnel: w33 -> [_ _ _ _ _ _ _]
    frame "invalid app kind", Default {
    }
    frame "Development System" {
      w490 = T13 5 items=["User Home"=0, "User Desktop"=1, "User Documents"=2, "User Application Data"=3, "User Preferences"=4, "User Temporary"=5, "Public Documents"=6, "Public Application Data"=7, "Public Preferences"=8, "Public Cache"=13, "System Core Libraries"=9, "System Installed Libraries"=10, "Application Files"=11, "Boot Volume Root"=12] ("system directory type")
      n250 = call <vilib>:"Get System Directory.vi"("create directory if not found? (F)"=TRUE, "system directory type"=w490) -> ("system directory"=w492:path)  [unwired: 9 in]
      n251 = Build Path(base path=w492, name or relative path="Archive and ftp") -> (appended path=w494:path)
      n252 = Delete(path (use dialog)=w494, entire hierarchy (F)=TRUE) -> (error out=w489:errorcluster)  [unwired: 3 in, 2 out]
      n253 = call <vilib>:"Clear Errors.vi"("error in (no error)"=w489) -> ()  [unwired: 6 in, 1 out]
    }
    frame "Run Time System" {
      n254 = flat-sequence {
        frame #0 {
          w497 = T13 5 items=["User Home"=0, "User Desktop"=1, "User Documents"=2, "User Application Data"=3, "User Preferences"=4, "User Temporary"=5, "Public Documents"=6, "Public Application Data"=7, "Public Preferences"=8, "Public Cache"=13, "System Core Libraries"=9, "System Installed Libraries"=10, "Application Files"=11, "Boot Volume Root"=12] ("system directory type")
          n255 = call <vilib>:"Get System Directory.vi"("create directory if not found? (F)"=TRUE, "system directory type"=w497) -> ("system directory"=w499:path)  [unwired: 9 in]
          n256 = Build Path(base path=w499, name or relative path="Archive and ftp") -> (appended path=w501:path)
          n257 = Delete(path (use dialog)=w501, entire hierarchy (F)=TRUE) -> (error out=w496:errorcluster)  [unwired: 3 in, 2 out]
          n258 = call <vilib>:"Clear Errors.vi"("error in (no error)"=w496) -> ()  [unwired: 6 in, 1 out]
        }
        frame #1 {
          n259 = Quit LabVIEW() -> ()  [unwired: 1 in]
        }
      }
    }
    frame "Student Edition" {
    }
    frame "Embedded LabVIEW" {
    }
    frame "Evaluation" {
    }
    frame "Custom" {
    }
  }
